vi "GetParameterList.vi"(8 "error in (no error)":errorcluster, 11 "ZWO_ASI in":refnum<class "ZWO_ASI.lvclass">) -> (0 "error out":errorcluster, 2 "Parameter List":T1(array[cluster]), 3 "ZWO_ASI out":refnum<class "ZWO_ASI.lvclass">)   [LabVIEW 2023, in "ZWO_ASI.lvlib" / "ZWO_ASI.lvclass"]
uses:
  ZWO_ASI.lvclass
  ZWO_ASI.lvclass/ZWO_ASI.ctl
  <userlib>/ASICamera2_no_err/ASICamera2_no_err.lvlib
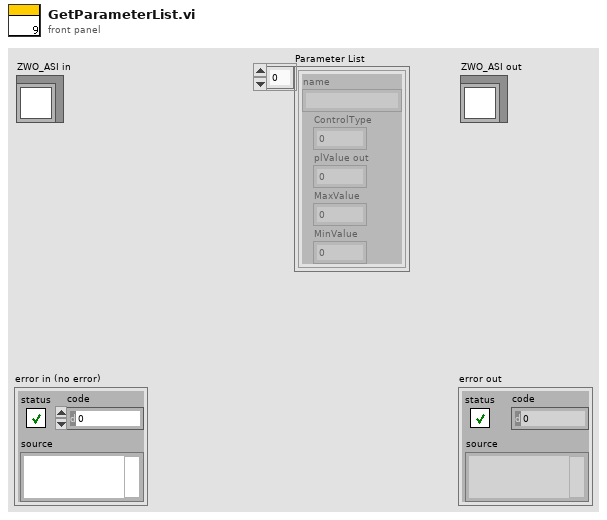
[diagram p1: front panel]
types:
  T1 = cluster{"name":string, "ControlType":u32, "plValue out":i32, "MaxValue":i32, "MinValue":i32}[]
  T2 = cluster{"Name[0]":i8, "Name[1]":i8, "Name[2]":i8, "Name[3]":i8, "Name[4]":i8, "Name[5]":i8, "Name[6]":i8, "Name[7]":i8, "Name[8]":i8, "Name[9]":i8, "Name[10]":i8, "Name[11]":i8, "Name[12]":i8, "Name[13]":i8, "Name[14]":i8, "Name[15]":i8, "Name[16]":i8, "Name[17]":i8, "Name[18]":i8, "Name[19]":i8, "Name[20]":i8, "Name[21]":i8, "Name[22]":i8, "Name[23]":i8, "Name[24]":i8, "Name[25]":i8, "Name[26]":i8, "Name[27]":i8, "Name[28]":i8, "Name[29]":i8, "Name[30]":i8, "Name[31]":i8, "Name[32]":i8, "Name[33]":i8, "Name[34]":i8, "Name[35]":i8, "Name[36]":i8, "Name[37]":i8, "Name[38]":i8, "Name[39]":i8, "Name[40]":i8, "Name[41]":i8, "Name[42]":i8, "Name[43]":i8, "Name[44]":i8, "Name[45]":i8, "Name[46]":i8, "Name[47]":i8, "Name[48]":i8, "Name[49]":i8, "Name[50]":i8, "Name[51]":i8, "Name[52]":i8, "Name[53]":i8, "Name[54]":i8, "Name[55]":i8, "Name[56]":i8, "Name[57]":i8, "Name[58]":i8, "Name[59]":i8, "Name[60]":i8, "Name[61]":i8, "Name[62]":i8, "Name[63]":i8, "Description[0]":i8, "Description[1]":i8, "Description[2]":i8, "Description[3]":i8, "Description[4]":i8, "Description[5]":i8, "Description[6]":i8, "Description[7]":i8, "Description[8]":i8, "Description[9]":i8, "Description[10]":i8, "Description[11]":i8, "Description[12]":i8, "Description[13]":i8, "Description[14]":i8, "Description[15]":i8, "Description[16]":i8, "Description[17]":i8, "Description[18]":i8, "Description[19]":i8, "Description[20]":i8, "Description[21]":i8, "Description[22]":i8, "Description[23]":i8, "Description[24]":i8, "Description[25]":i8, "Description[26]":i8, "Description[27]":i8, "Description[28]":i8, "Description[29]":i8, "Description[30]":i8, "Description[31]":i8, "Description[32]":i8, "Description[33]":i8, "Description[34]":i8, "Description[35]":i8, "Description[36]":i8, "Description[37]":i8, "Description[38]":i8, "Description[39]":i8, "Description[40]":i8, "Description[41]":i8, "Description[42]":i8, "Description[43]":i8, "Description[44]":i8, "Description[45]":i8, "Description[46]":i8, "Description[47]":i8, "Description[48]":i8, "Description[49]":i8, "Description[50]":i8, "Description[51]":i8, "Description[52]":i8, "Description[53]":i8, "Description[54]":i8, "Description[55]":i8, "Description[56]":i8, "Description[57]":i8, "Description[58]":i8, "Description[59]":i8, "Description[60]":i8, "Description[61]":i8, "Description[62]":i8, "Description[63]":i8, "Description[64]":i8, "Description[65]":i8, "Description[66]":i8, "Description[67]":i8, "Description[68]":i8, "Description[69]":i8, "Description[70]":i8, "Description[71]":i8, "Description[72]":i8, "Description[73]":i8, "Description[74]":i8, "Description[75]":i8, "Description[76]":i8, "Description[77]":i8, "Description[78]":i8, "Description[79]":i8, "Description[80]":i8, "Description[81]":i8, "Description[82]":i8, "Description[83]":i8, "Description[84]":i8, "Description[85]":i8, "Description[86]":i8, "Description[87]":i8, "Description[88]":i8, "Description[89]":i8, "Description[90]":i8, "Description[91]":i8, "Description[92]":i8, "Description[93]":i8, "Description[94]":i8, "Description[95]":i8, "Description[96]":i8, "Description[97]":i8, "Description[98]":i8, "Description[99]":i8, "Description[100]":i8, "Description[101]":i8, "Description[102]":i8, "Description[103]":i8, "Description[104]":i8, "Description[105]":i8, "Description[106]":i8, "Description[107]":i8, "Description[108]":i8, "Description[109]":i8, "Description[110]":i8, "Description[111]":i8, "Description[112]":i8, "Description[113]":i8, "Description[114]":i8, "Description[115]":i8, "Description[116]":i8, "Description[117]":i8, "Description[118]":i8, "Description[119]":i8, "Description[120]":i8, "Description[121]":i8, "Description[122]":i8, "Description[123]":i8, "Description[124]":i8, "Description[125]":i8, "Description[126]":i8, "Description[127]":i8, "MaxValue":i32, "MinValue":i32, "DefaultValue":i32, "IsAutoSupported":u32, "IsWritable":u32, "ControlType":u32, "Unused[0]":i8, "Unused[1]":i8, "Unused[2]":i8, "Unused[3]":i8, "Unused[4]":i8, "Unused[5]":i8, "Unused[6]":i8, "Unused[7]":i8, "Unused[8]":i8, "Unused[9]":i8, "Unused[10]":i8, "Unused[11]":i8, "Unused[12]":i8, "Unused[13]":i8, "Unused[14]":i8, "Unused[15]":i8, "Unused[16]":i8, "Unused[17]":i8, "Unused[18]":i8, "Unused[19]":i8, "Unused[20]":i8, "Unused[21]":i8, "Unused[22]":i8, "Unused[23]":i8, "Unused[24]":i8, "Unused[25]":i8, "Unused[26]":i8, "Unused[27]":i8, "Unused[28]":i8, "Unused[29]":i8, "Unused[30]":i8, "Unused[31]":i8}
  T3 = cluster{"name":string, "ControlType":u32, "plValue out":i32, "MaxValue":i32, "MinValue":i32}
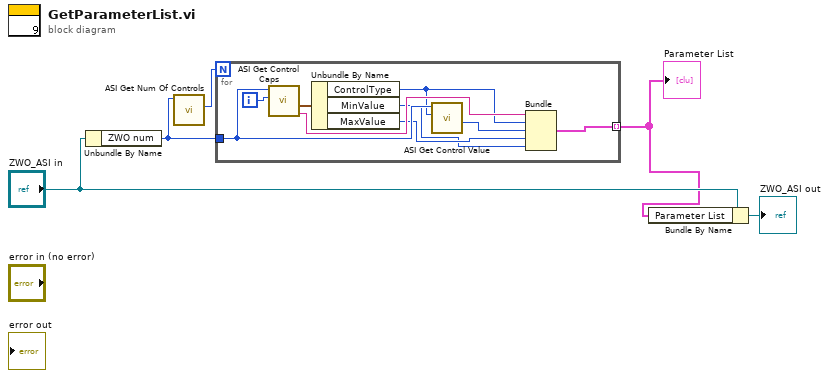
[diagram p0: block diagram]
diagram:
  n1 = Unbundle By Name("ZWO_ASI in") -> ("ZWO num"=w4:i32)
  n2 = call <userlib>:"ASI Get Num Of Controls.vi"("iCameraID"=w4) -> ("piNumberOfControls out"=w5:i32)  [unwired: 9 in, 1 out]
  n3 = for {
    N: w5 -> [_]
    tunnel: w4 -> [w14]
    tunnel: [w10] -> w1 mode=indexing
    i -> [w13]
    n4 = call <userlib>:"ASI Get Control Caps.vi"("iControlIndex"=w13, "iCameraID"=w14) -> ("name"=w12:string, "pControlCaps out"=w11:T2)  [unwired: 7 in, 1 out]
    n5 = Unbundle By Name(w11) -> ("ControlType"=w8:u32, "MinValue"=w6:i32, "MaxValue"=w9:i32)
    n6 = call <userlib>:"ASI Get Control Value.vi"("ControlType"=w8, "iCameraID"=w14) -> ("plValue out"=w7:i32)  [unwired: 7 in, 2 out]
    n7 = Bundle("name"=w12, "ControlType"=w8, "plValue out"=w7, "MaxValue"=w9, "MinValue"=w6) -> (w10:T3)  [unwired: 1 in]
  }
  "Parameter List" <- w1
  n8 = Bundle By Name(cluster="ZWO_ASI in", "Parameter List"=w1) -> (→"ZWO_ASI out":refnum<class "ZWO_ASI.lvclass">)
